vi "Load Auton by Name.vi"(11 "String":string) -> (0 "error out":errorcluster, 3 "Auton Sequence":T1[](array[typedef]))   [LabVIEW 2017]
uses:
  AutonBuilder/Typedef/Single Sequence.ctl
  AutonBuilder/Typedef/Sequence Command.ctl
  AutonBuilder/Typedef/Plate Arrangement.ctl
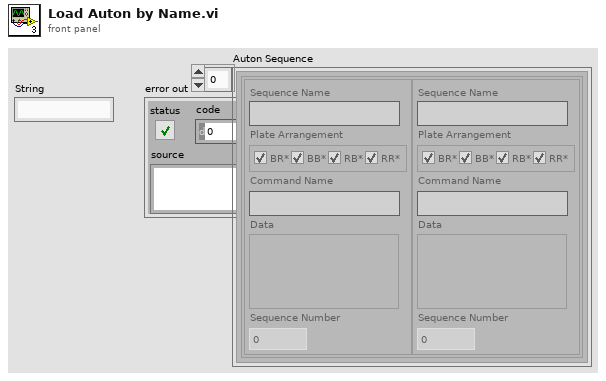
[diagram p1: front panel]
types:
  T1 = typedef "Single Sequence.ctl" = cluster{"Sequence Array":T2[]}
  T2 = typedef "Sequence Command.ctl" = cluster{"Sequence Name":string, "Plate Arrangement":T3, "Command Name":string, "Data":variant, "Sequence Number":u32}
  T3 = typedef "Plate Arrangement.ctl" = cluster{"BR*":bool, "BB*":bool, "RB*":bool, "RR*":bool}
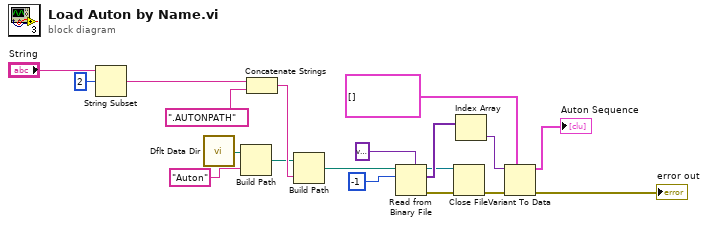
[diagram p0: block diagram]
diagram:
  n1 = String Subset(string="String", offset (0)=2) -> (substring=w1:string)  [unwired: 1 in]
  n2 = call <vilib>:"Dflt Data Dir.vi"() -> ("App:Default Data Directory"=w15:path)
  n3 = Build Path(base path=w15, name or relative path="Auton") -> (appended path=w17:path)
  n4 = Concatenate Strings(w1, ".AUTONPATH" ("string")) -> (w18:string)
  n5 = Build Path(base path=w17, name or relative path=w18) -> (appended path=w19:path)
  n6 = Read from Binary File(5:variant, 10:-1 ("count (1)"), 11:w19) -> (0:w5:errorcluster, 2:w9:variant[], 3:w6:refnum<file>)  [unwired: 3 in, 1 out]
  n7 = Close File(refnum=w6, error in=w5) -> (error out=w8:errorcluster)  [unwired: 1 out]
  n8 = Index Array(array=w9) -> (element=w10:variant)  [unwired: 1 in]
  n9 = Variant To Data(error in=w8, type=T1[] [] ("Auton Sequence"), Variant=w10) -> (data=→"Auton Sequence":T1[], error out=→"error out":errorcluster)
